vi "Teardown.vi"(11 "Queue Transport in":refnum<class "Queue Transport.lvclass">) -> (2 "Unhandled Msgs":refnum<class "Msg.lvclass">[](array[class]))   [LabVIEW 2025, in "jettl.lvlib" / "Transport.lvlib" / "Queue.lvlib" / "Queue Transport.lvclass"]
uses:
  Queue Transport.lvclass
  Msg/Msg.lvclass
  Queue Transport.lvclass/Queue Transport.ctl
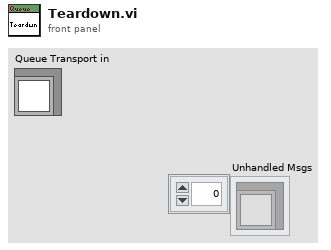
[diagram p1: front panel]
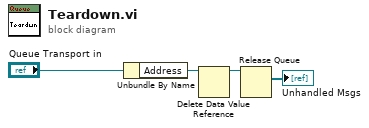
[diagram p0: block diagram]
diagram:
  n1 = Unbundle By Name("Queue Transport in") -> ("Address"=w2:refnum<data-value>)
  n2 = Delete Data Value Reference(data value reference=w2) -> (data value=w1:refnum<queue>)  [unwired: 1 in, 1 out]
  n3 = Release Queue(queue=w1) -> (remaining elements=→"Unhandled Msgs":refnum<class "Msg.lvclass">[])  [unwired: 2 in, 2 out]
